vi "Write Message Icon.vi"(10 "Message Icon":refnum<class "Icon.lvclass">, 11 "Message Scripter in":refnum<class "Message Scripter.lvclass">) -> (3 "Message Scripter out":refnum<class "Message Scripter.lvclass">)   [LabVIEW 2020, in "Message Maker.lvlib" / "Message Scripter.lvclass"]
uses:
  Message Scripter.lvclass
  <vilib>/LabVIEW Icon API/lv_icon/Classes/Icon/Icon.lvclass
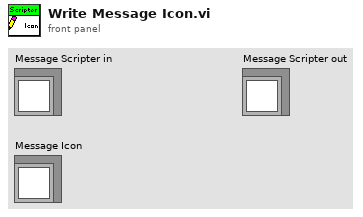
[diagram p1: front panel]
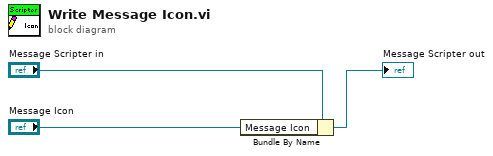
[diagram p0: block diagram]
diagram:
  n1 = Bundle By Name(cluster="Message Scripter in", "Message Icon"="Message Icon") -> (→"Message Scripter out":refnum<class "Message Scripter.lvclass">)
